vi "test Get Attribute as DBL.vi"(11 "Test Case In":refnum<class "Test Config From EXCEL.lvclass">) -> (0 "error out":errorcluster, 3 "Test Case Out":refnum<class "Test Config From EXCEL.lvclass">)   [LabVIEW 2020, in "Test Config From EXCEL.lvclass"]
uses:
  Test Config From EXCEL.lvclass
  Test Config From EXCEL.lvclass/Test Config From EXCEL.ctl
  Source/Config from EXCEL/Config from EXCEL.lvclass
  <vilib>/Astemes/LUnit/Test Case.lvclass
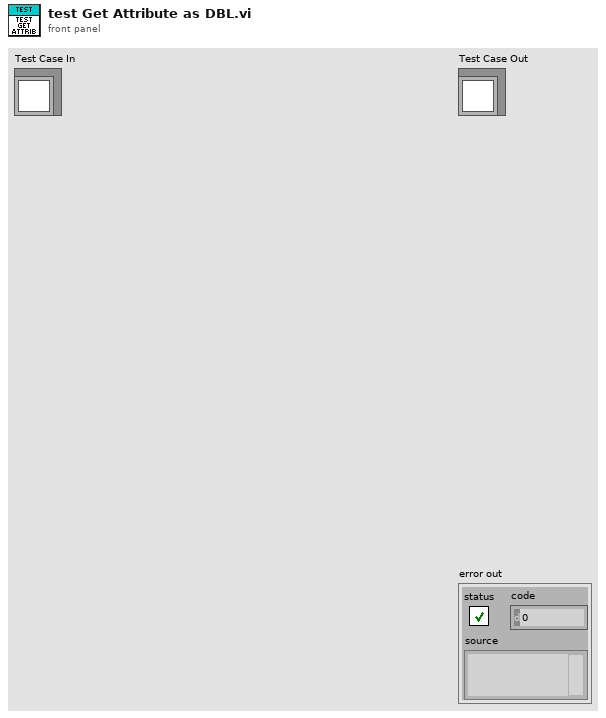
[diagram p1: front panel]
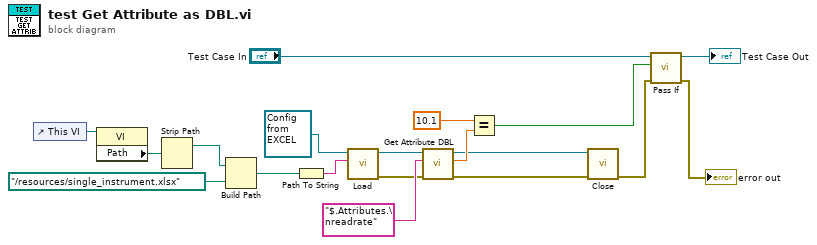
[diagram p0: block diagram]
diagram:
  n1 = control-ref of="This VI"() -> (w13:refnum<vi>)
  n2 = property class="VI"(reference=w13) -> ("Path"=w12:path)  [unwired: 1 in, 2 out]
  n3 = Strip Path(path=w12) -> (stripped path=w10:path)  [unwired: 1 out]
  n4 = Build Path(base path=w10, name or relative path=path "../resources/single_instrument.xlsx") -> (appended path=w11:path)
  n5 = Path To String(path=w11) -> (string=w14:string)
  n6 = call-dynamic "Load.vi"("Source"=w14, "Config from EXCEL in"=refnum<class "Config from EXCEL.lvclass"> refnum ("Config from EXCEL.lvclass")) -> ("error out"=w1:errorcluster, "Config from EXCEL out"=w2:refnum<class "Config from EXCEL.lvclass">)  [unwired: 8 in]
  n7 = call-dynamic "Get Attribute DBL.vi"("error in"=w1, "Attribute"="$.Attributes.\nreadrate", "Config from EXCEL in"=w2) -> ("error out"=w4:errorcluster, "Value"=w7:dbl, "Config from EXCEL out"=w5:refnum<class "Config from EXCEL.lvclass">)  [unwired: 6 in]
  n8 = Equal?(x=10.1 ("Value"), y=w7) -> (x = y?=w6:bool)
  n9 = call-dynamic "Close.vi"("error in"=w4, "Config from EXCEL in"=w5) -> ("error out"=w3:errorcluster)  [unwired: 8 in, 1 out]
  n10 = call <vilib>:"Pass If.vi"("error in (no error)"=w3, "Pass?"=w6, "LUnit Test Case In"="Test Case In") -> ("error out"=→"error out":errorcluster, "LUnit Test Case Out"=→"Test Case Out":refnum<class "Test Config From EXCEL.lvclass">)  [unwired: 7 in]
